vi "solar_log New File.vi"(4 "Pending (0)":i32, 6 "Backlog (0)":i32, 8 "error in (no error)":errorcluster, 10 "LogsDir":path, 11 "Old FileRefnum in":refnum<file>) -> (0 "error out":errorcluster, 2 "LogPath":path, 3 "New FileRefnum out":refnum<file>)   [LabVIEW 2018]
doc: "This creates a new log file. The current time is used to uniquely identify the filename."
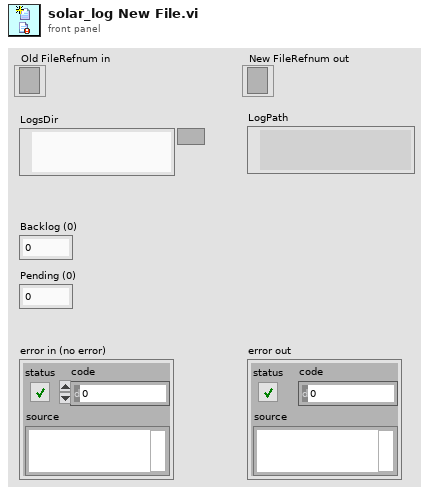
[diagram p1: front panel]
types:
  T1 = enum16{"open", "replace", "create", "open or create", "replace or create", "replace or create with confirmation"}
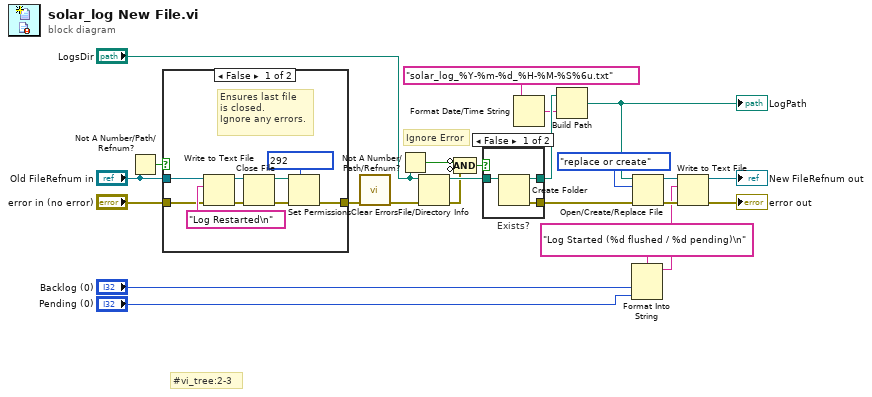
[diagram p0: block diagram]
diagram:
  # "#vi_tree:2-3"
  # "Ignore Error"
  n1 = Not A Number/Path/Refnum?(number/path/refnum="Old FileRefnum in") -> (NaN/Path/Refnum?=w5:bool)
  n2 = case shown="False" w5 {
    tunnel: [w33 w34] -> w23
    tunnel: "error in (no error)" -> [w26 w34]
    tunnel: "Old FileRefnum in" -> [w25 _]
    frame False {
      # "Ensures last file\nis closed.\nIgnore any errors."
      n3 = Write to Text File(file (use dialog)=w25, text="Log Restarted\n", error in=w26) -> (refnum out=w31:refnum<file>, error out=w30:errorcluster)  [unwired: 1 in, 1 out]
      n4 = Close File(refnum=w31, error in=w30) -> (path=w28:path, error out=w29:errorcluster)
      n5 = Set Permissions(7:i16 292 ("permissions"), 8:w29, 11:w28) -> (0:w33:errorcluster)  [unwired: 2 in, 1 out]
    }
    frame True {
      # "Invalid refnum"
    }
  }
  n6 = call <vilib>:"Clear Errors.vi"("error in (no error)"=w23) -> ("error out"=w24:errorcluster)  [unwired: 5 in, 1 out]
  n7 = Not A Number/Path/Refnum?(number/path/refnum="LogsDir") -> (NaN/Path/Refnum?=w15:bool)
  n8 = File/Directory Info(path="LogsDir", error in=w24) -> (path out=w18:path, error out=w16:errorcluster)  [unwired: 5 out]
  n9 = Compound Arithmetic op=AND(invert w15, invert w16) -> (w17:bool)
  n10 = case "Exists?" shown="False" w17 {
    tunnel: w18 -> [w37 w38]
    tunnel: [w36 _] -> w11
    tunnel: [w35 w38] -> w10
    frame False {
      n11 = Create Folder(path (use dialog)=w37) -> (created path=w35:path, error out=w36:errorcluster)  [unwired: 2 in, 1 out]
    }
    frame True {
    }
  }
  n12 = Format Date/Time String(time format string (%c)="solar_log_%Y-%m-%d_%H-%M-%S%6u.txt" ("format string")) -> (date/time string=w8:string)  [unwired: 2 in]
  n13 = Build Path(base path=w10, name or relative path=w8) -> (appended path=w20:path)
  "LogPath" <- w20
  n14 = Format Into String(format string="Log Started (%d flushed / %d pending)\n" ("text"), "Backlog (0)", "Pending (0)") -> (resulting string=w2:string)  [unwired: 2 in, 1 out]
  n15 = Open/Create/Replace File(file path (use dialog)=w20, error in=w11, operation (0:open)=T1."replace or create") -> (refnum out=w13:refnum<file>, error out=w12:errorcluster)  [unwired: 3 in, 1 out]
  n16 = Write to Text File(file (use dialog)=w13, text=w2, error in=w12) -> (refnum out=→"New FileRefnum out":refnum<file>, error out=→"error out":errorcluster)  [unwired: 1 in, 1 out]
